vi "Convert to 180.vi"(1 "Angle In":dbl) -> (0 "Angle Out":dbl)   [LabVIEW 2015]
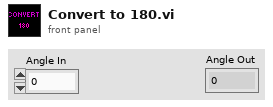
[diagram p1: front panel]
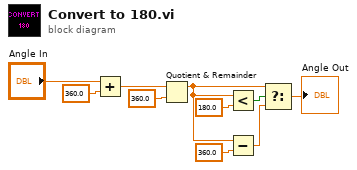
[diagram p0: block diagram]
diagram:
  n1 = Add(x="Angle In", y=360.0) -> (x+y=w8:dbl)
  n2 = Quotient & Remainder(x=w8, y=360.0) -> (x-y*floor(x/y)=w3:dbl)  [unwired: 1 out]
  n3 = Less?(x=w3, y=180.0) -> (x < y?=w4:bool)
  n4 = Subtract(x=w3, y=360.0) -> (x-y=w1:dbl)
  n5 = Select(t=w3, s=w4, f=w1) -> (s? t:f=→"Angle Out":dbl)
